vi "Facade.vi"(0 "Data In":T5, 2 "Display State In":T2, 3 "Container State":T4) -> (6 "Data Out":T5, 7 "Display State Out":T2, 8 "Action":T1)   [LabVIEW 2015, in "Noise (G3).xctl"]
uses:
  Noise (G3).xctl
  Data.ctl
  <vilib>/_xctls/Container State.ctl
  State.ctl
  Noise (G3) - Persistent.ctl
  <vilib>/_xctls/Action.ctl
  <vilib>/_xctls/XControlSupport.lvlib
panel:
  in  "Brickwall":bool
  out "display state signal":bool
  in  "Inverse filter":bool caption="Acoustic system compensation"
  in  "A-weight":bool caption="Audiogram compensation"
  in  "Seed":i32
  in  "Tokens":i32 min=0 step=1
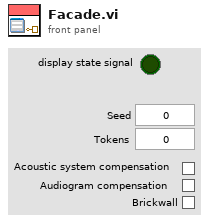
[diagram p1: front panel]
types:
  T1 = typedef "XControlSupport.lvlib/Action.ctl" = cluster{"Data Changed?":bool, "State Changed?":bool, "Action Name":string}
  T2 = typedef "Noise (G3).xctl/State.ctl" = cluster{"enable menu":bool, "persistent":T3}
  T3 = typedef "Noise (G3).xctl/Noise (G3) - Persistent.ctl" = cluster{"Show Aweight":bool}
  T4 = typedef "XControlSupport.lvlib/Container State.ctl" = cluster{"Indicator?":bool, "Run Mode?":bool, " Refnum":refnum<vi>}
  T5 = typedef "Noise (G3).xctl/Data.ctl" = cluster{"InvFilt":bool, "Aweight":bool, "Seed":i32, "Tokens":i32, "Brickwall":bool}
  T6 = enum8{"Enabled", "Disabled", "Disabled and Grayed Out"}
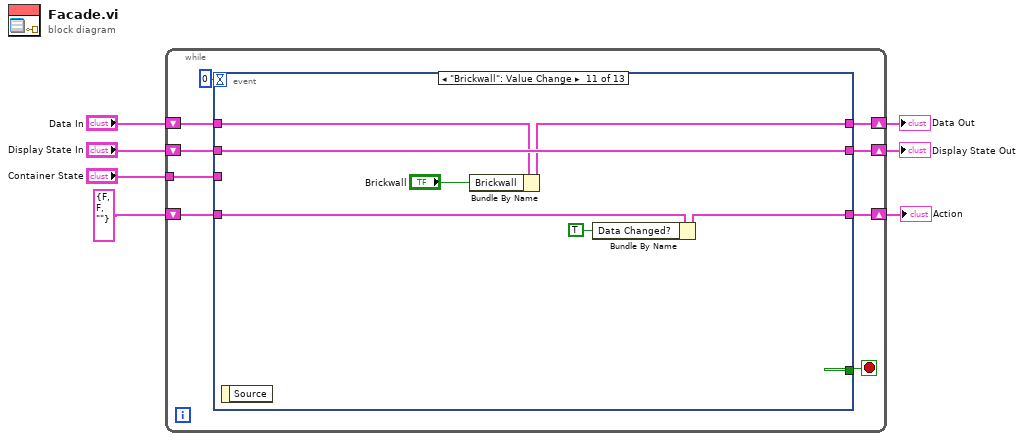
[diagram p0: block diagram]
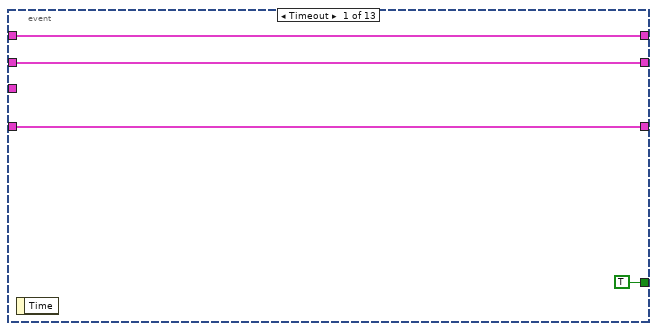
[diagram p2: hidden frame]
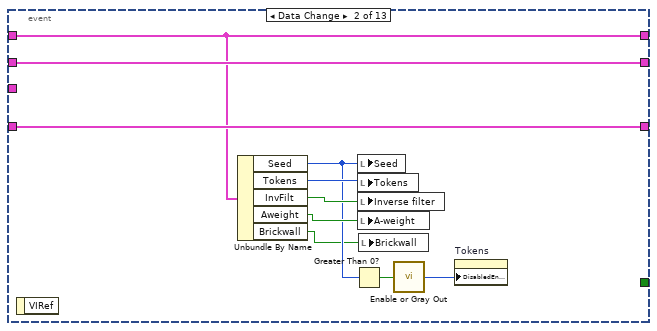
[diagram p3: hidden frame]
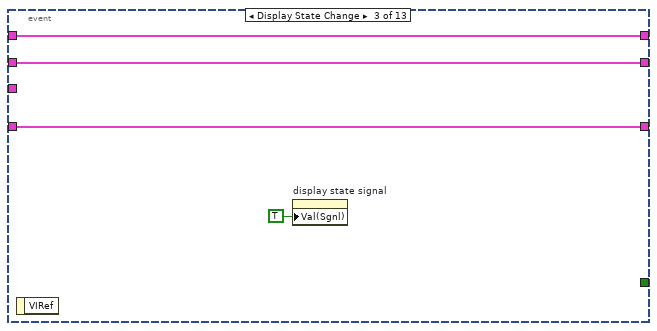
[diagram p4: hidden frame]
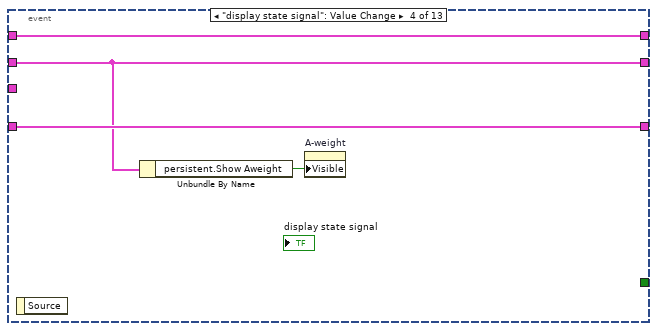
[diagram p5: hidden frame]
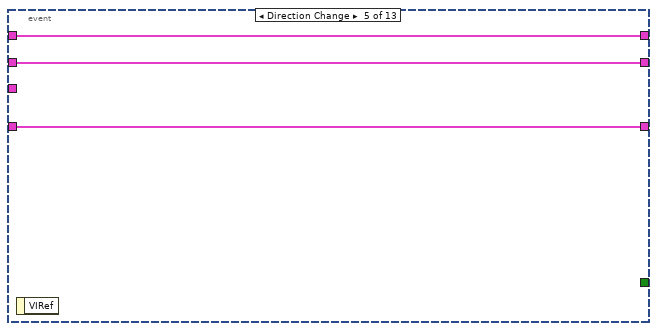
[diagram p6: hidden frame]
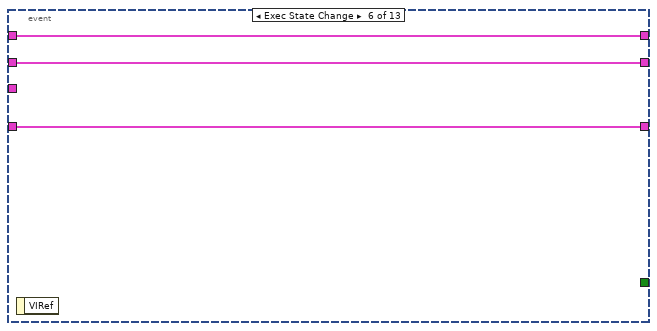
[diagram p7: hidden frame]
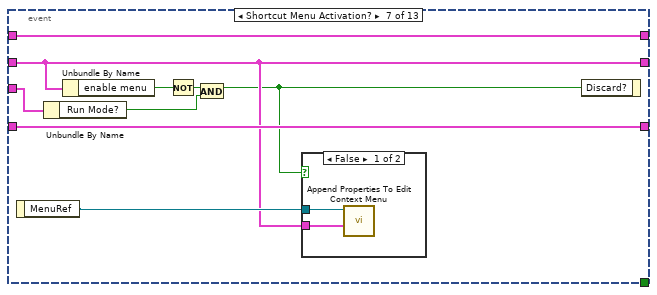
[diagram p8: hidden frame]
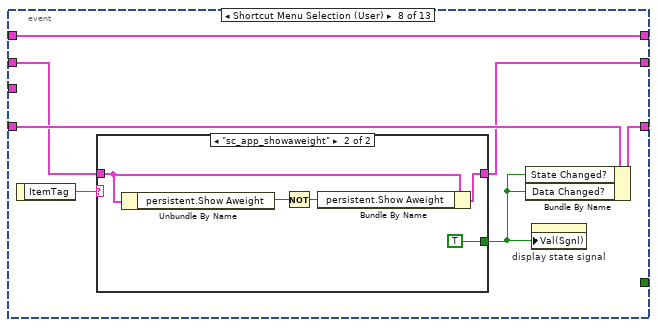
[diagram p10: hidden frame]
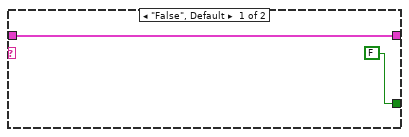
[diagram p11: hidden frame]
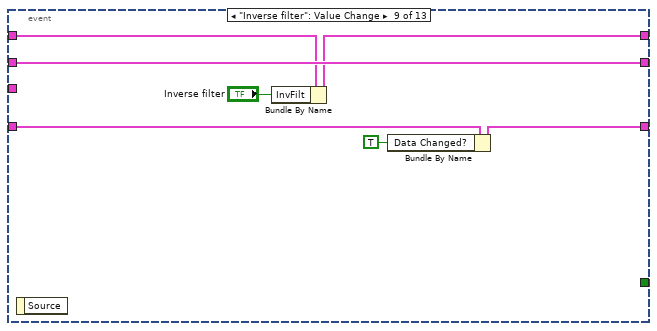
[diagram p12: hidden frame]
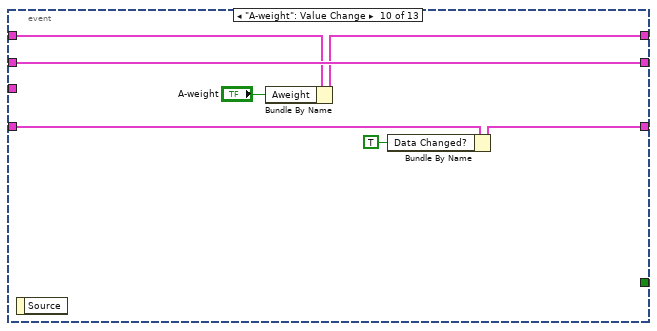
[diagram p13: hidden frame]
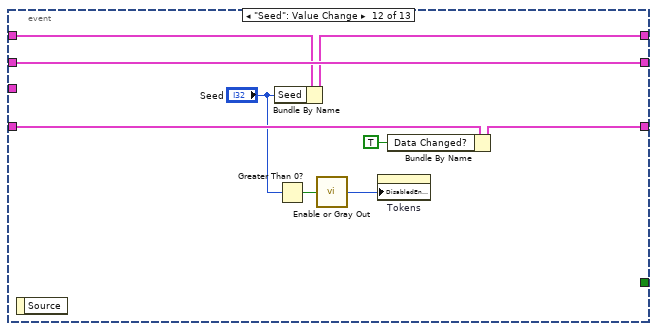
[diagram p14: hidden frame]
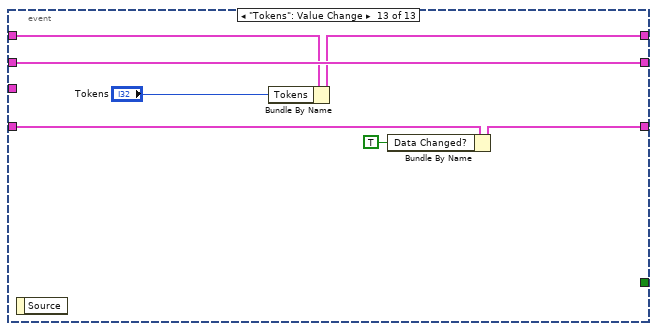
[diagram p15: hidden frame]
diagram:
  n1 = while {
    shift-right: [w15] -> w4
    shift-left: "Display State In" -> [w16]
    tunnel: "Container State" -> [w12]
    shift-right: [w10] -> w7
    shift-left: "Data In" -> [w11]
    shift-right: [w8] -> w2
    shift-left: T1 {"Data Changed?"=FALSE, "State Changed?"=FALSE, "Action Name"=""} ("Action") -> [w9]
    stop <- w14 stop-if-true
    n2 = event shown="[10] \"Brickwall\": Value Change" {
      selector: _ -> [_ _ _ _ _ _ _ _ _ _ _ _ _]
      dyn-events: _ -> [_ _ _ _ _ _ _ _ _ _ _ _ _]
      timeout: 0 -> [_ _ _ _ _ _ _ _ _ _ _ _ _]
      tunnel: w16 -> [w18 w30 w32 w36 w41 w44 w50 w59 w76 w83 w90 w99 w106]
      tunnel: [w18 w30 w32 w36 w41 w44 w50 w58 w76 w83 w90 w99 w106] -> w15
      tunnel: [TRUE _ _ _ _ _ _ _ _ _ _ _ _] -> w14
      tunnel: w12 -> [_ _ _ _ _ _ w48 _ _ _ _ _ _]
      tunnel: w11 -> [w17 w28 w34 w38 w40 w43 w53 w57 w75 w82 w89 w98 w105]
      tunnel: [w17 w28 w34 w38 w40 w43 w53 w57 w73 w80 w87 w96 w103] -> w10
      tunnel: [w19 w29 w33 w37 w39 w42 w52 w60 w71 w79 w86 w95 w102] -> w8
      tunnel: w9 -> [w19 w29 w33 w37 w39 w42 w52 w62 w74 w81 w88 w97 w104]
      event Timeout {
        n3 = event-data() -> ()  [unwired: 1 in, 1 out]
      }
      event Data Change {
        n4 = event-data() -> ()  [unwired: 1 in, 1 out]
        n5 = Unbundle By Name(w28) -> ("Seed"=w23:i32, "Tokens"=w27:i32, "InvFilt"=w26:bool, "Aweight"=w25:bool, "Brickwall"=w21:bool)
        n6 = Greater Than 0?(x=w23) -> (x > 0?=w22:bool)
        n7 = local write "Seed"(w23) -> ()
        n8 = local write "Tokens"(w27) -> ()
        n9 = local write "Inverse filter"(w26) -> ()
        n10 = local write "A-weight"(w25) -> ()
        n11 = local write "Brickwall"(w21) -> ()
        n12 = call "Enable or Gray Out.vi"("Boolean"=w22) -> ("Disabled"=w24:T6)
        n13 = property on="Tokens" class="DigNum (strict)"("DisabledEnum"=w24) -> ()  [unwired: 2 in, 2 out]
      }
      event Display State Change {
        n14 = event-data() -> ()  [unwired: 1 in, 1 out]
        n15 = property on="display state signal" class="Bool (strict)"("Val(Sgnl)"=TRUE ("Value (Signaling)")) -> ()  [unwired: 2 in, 2 out]
      }
      event "display state signal": Value Change {
        n16 = event-data() -> ()  [unwired: 1 in, 1 out]
        n17 = Unbundle By Name(w36) -> ("persistent.Show Aweight"=w35:bool)
        n18 = property on="A-weight" class="Bool (strict)"("Visible"=w35) -> ()  [unwired: 2 in, 2 out]
      }
      event Direction Change {
        n19 = event-data() -> ()  [unwired: 1 in, 1 out]
      }
      event Exec State Change {
        n20 = event-data() -> ()  [unwired: 1 in, 1 out]
      }
      event Shortcut Menu Activation? {
        n21 = event-data() -> ("MenuRef"=w51:refnum<k9>)  [unwired: 1 in]
        n22 = Unbundle By Name(w48) -> ("Run Mode?"=w46:bool)
        n23 = Unbundle By Name(w50) -> ("enable menu"=w45:bool)
        n24 = Not(x=w45) -> (.not. x?=w47:bool)
        n25 = And(x=w47, y=w46) -> (x .and. y?=w49:bool)
        n26 = case shown="False" w49 {
          tunnel: w51 -> [w55 _]
          tunnel: w50 -> [w54 _]
          frame False {
            n27 = call "Append Properties To Edit Context Menu.vi"("State"=w54, "Menu in"=w55) -> ()  [unwired: 10 in]
          }
          frame True {
          }
        }
        n28 = event-data("Discard?"=w49) -> ()  [unwired: 1 in, 1 out]
      }
      event Shortcut Menu Selection (User) {
        n29 = event-data() -> ("ItemTag"=w61:string)  [unwired: 1 in]
        n30 = case shown="\"sc_app_showaweight\"" w61 {
          tunnel: w59 -> [w64 w68]
          tunnel: [w64 w67] -> w58
          tunnel: [FALSE TRUE] -> w56
          frame "False", Default {
          }
          frame "sc_app_showaweight" {
            n31 = Unbundle By Name(w68) -> ("persistent.Show Aweight"=w66:bool)
            n32 = Not(x=w66) -> (.not. x?=w65:bool)
            n33 = Bundle By Name(cluster=w68, "persistent.Show Aweight"=w65) -> (w67:T2)
          }
        }
        n34 = Bundle By Name(cluster=w62, "State Changed?"=w56, "Data Changed?"=w56) -> (w60:T1)
        n35 = property on="display state signal" class="Bool (strict)"("Val(Sgnl)"=w56) -> ()  [unwired: 2 in, 2 out]
      }
      event "Inverse filter": Value Change {
        n36 = event-data() -> ()  [unwired: 1 in, 1 out]
        n37 = Bundle By Name(cluster=w75, "InvFilt"="Inverse filter") -> (w73:T5)
        n38 = Bundle By Name(cluster=w74, "Data Changed?"=TRUE) -> (w71:T1)
      }
      event "A-weight": Value Change {
        n39 = event-data() -> ()  [unwired: 1 in, 1 out]
        n40 = Bundle By Name(cluster=w82, "Aweight"="A-weight") -> (w80:T5)
        n41 = Bundle By Name(cluster=w81, "Data Changed?"=TRUE) -> (w79:T1)
      }
      event "Brickwall": Value Change {
        n42 = event-data() -> ()  [unwired: 1 in, 1 out]
        n43 = Bundle By Name(cluster=w89, "Brickwall"="Brickwall") -> (w87:T5)
        n44 = Bundle By Name(cluster=w88, "Data Changed?"=TRUE) -> (w86:T1)
      }
      event "Seed": Value Change {
        n45 = event-data() -> ()  [unwired: 1 in, 1 out]
        n46 = Bundle By Name(cluster=w98, "Seed"="Seed") -> (w96:T5)
        n47 = Greater Than 0?(x="Seed") -> (x > 0?=w92:bool)
        n48 = call "Enable or Gray Out.vi"("Boolean"=w92) -> ("Disabled"=w91:T6)
        n49 = property on="Tokens" class="DigNum (strict)"("DisabledEnum"=w91) -> ()  [unwired: 2 in, 2 out]
        n50 = Bundle By Name(cluster=w97, "Data Changed?"=TRUE) -> (w95:T1)
      }
      event "Tokens": Value Change {
        n51 = event-data() -> ()  [unwired: 1 in, 1 out]
        n52 = Bundle By Name(cluster=w105, "Tokens"="Tokens") -> (w103:T5)
        n53 = Bundle By Name(cluster=w104, "Data Changed?"=TRUE) -> (w102:T1)
      }
    }
  }
  "Display State Out" <- w4
  "Data Out" <- w7
  "Action" <- w2
